vi "Cleanup.vi"(11 "Timeout (-1)":i32) -> (0 "error out":errorcluster, 3 "WebFrontPanels":refnum<class "Web Front Panel.lvclass">[](array[class]))   [LabVIEW 2015, in "Front Panel Publisher.lvlib" / "Front Panel Manager.lvclass"]
uses:
  Front Panel Manager.lvclass
  Web Front Panel_class/Web Front Panel.lvclass
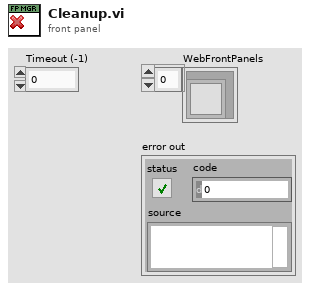
[diagram p1: front panel]
types:
  T1 = typedef "Front Panel Publisher.lvlib/Front Panel Manager.lvclass/Object Attributes.ctl" = cluster{"WebFrontPanels":refnum<class "Web Front Panel.lvclass">[], "WFP Names":string[], "Root folder":path, "Websocket Info":T2}
  T2 = typedef "Front Panel Publisher.lvlib/Front Panel Manager.lvclass/Websocket Info.ctl" = cluster{"Hostname":string, "Port":u16}
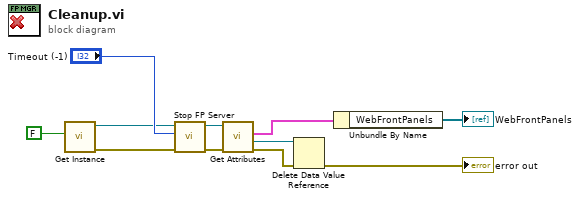
[diagram p0: block diagram]
diagram:
  n1 = call "Get Instance.vi"("Create If Not Exist (T)"=FALSE) -> ("error out"=w7:errorcluster, "FP Manager Out"=w6:refnum<class "Front Panel Manager.lvclass">)  [unwired: 6 in, 3 out]
  n2 = call "Stop FP Server.vi"("error in (no error)"=w7, "Timeout (-1)"="Timeout (-1)", "FP Management In"=w6) -> ("error out"=w8:errorcluster, "FP Management Out"=w9:refnum<class "Front Panel Manager.lvclass">)  [unwired: 7 in]
  n3 = call "Get Attributes.vi"("error in (no error)"=w8, "FP Management In"=w9) -> ("error out"=w2:errorcluster, "DataRef"=w3:refnum<data-value>, "Data"=w4:T1)  [unwired: 6 in, 1 out]
  n4 = Delete Data Value Reference(data value reference=w3, error in=w2) -> (error out=→"error out":errorcluster)  [unwired: 1 out]
  n5 = Unbundle By Name(w4) -> ("WebFrontPanels"=→"WebFrontPanels":refnum<class "Web Front Panel.lvclass">[])
